vi "Laser Power Control.vi"(7 "Calling VI Ref":refnum<vi>) -> ()   [LabVIEW 2020]
uses:
  Laser Power Control Type Defs/Laser Power Ctrl Main Control.ctl
  Laser Power Control Type Defs/Laser Power Ctrl Setup.ctl
  Hardware Configuration/Hardware Configuration Controls/Device Type.ctl
  <vilib>/Utility/miscctls.llb/LVPointTypeDef.ctl
  Laser Power Control Type Defs/Laser Power Ctrl Settings.ctl
  Hardware Configuration/Hardware Configuration Controls/Device Function.ctl
  Laser Power Control Type Defs/Laser Power Ctrl Notifier Type.ctl
  Laser Power Control Type Defs/Laser Power Ctrl Actions.ctl
  Laser Power Control Type Defs/Laser Power Ctrl Base Type.ctl
  Laser Power Control Type Defs/Laser Power Ctrl Type.ctl
  Device Library/Lasers/Laser Controls/Laser Actions.ctl
  Device Library/AOTFs/AOTF Controls/AOTF Actions.ctl
  Device Library/Lasers/External Power Control/External Power Control Type Defs/External Power Actions.ctl
  Device Manager/Common Device Queue/Common Device Controls/Common Device Actions.ctl
  <vilib>/regexp/Match Regular Expression.xnode
panel:
  in  "Manual Laser Ctrl.":bool
  out "Tab Control":enum32{"Power Adjust", "Setup"}(tab)
  in  "Power Ctrl 04":T1={"Wavelength (nm)"=0, "Active"=TRUE, "Power"=0.0, "Power Slider"=0, "Ctrl Status"=""} {"Power Slider" scale=0.0..100.0}
  in  "Power Ctrl 03":T1={"Wavelength (nm)"=0, "Active"=TRUE, "Power"=0.0, "Power Slider"=0, "Ctrl Status"=""} {"Power Slider" scale=0.0..100.0}
  in  "Power Ctrl 02":T1={"Wavelength (nm)"=0, "Active"=TRUE, "Power"=0.0, "Power Slider"=0, "Ctrl Status"=""} {"Power Slider" scale=0.0..100.0}
  in  "Power Ctrl 01":T1={"Wavelength (nm)"=0, "Active"=TRUE, "Power"=0.0, "Power Slider"=0, "Ctrl Status"=""} {"Power Slider" scale=0.0..100.0}
  in  "Power Ctrl 00":T1={"Wavelength (nm)"=0, "Active"=TRUE, "Power"=0.0, "Power Slider"=0, "Ctrl Status"=""} {"Power Slider" scale=0.0..100.0}
  in  "Power Setup 04":T2 {"Power Control Mode" items=["Direct", "AOTF", "External Ctrl", "Ext + AOTF"]}
  in  "Power Setup 03":T2 {"Power Control Mode" items=["Direct", "AOTF", "External Ctrl", "Ext + AOTF"]}
  in  "Power Setup 02":T2 {"Power Control Mode" items=["Direct", "AOTF", "External Ctrl", "Ext + AOTF"]}
  in  "Power Setup 01":T2 {"Power Control Mode" items=["Direct", "AOTF", "External Ctrl", "Ext + AOTF"]}
  in  "Power Setup 00":T2 {"Power Control Mode" items=["Direct", "AOTF", "External Ctrl", "Ext + AOTF"]}
  in  "Power Ctrl Setup":bool=TRUE
  in  "Quit":bool
  # "Ctrl Status:"
  # "Ctrl Status:"
  # "Ctrl Status:"
  # "Ctrl Status:"
  # "Ctrl Status:"
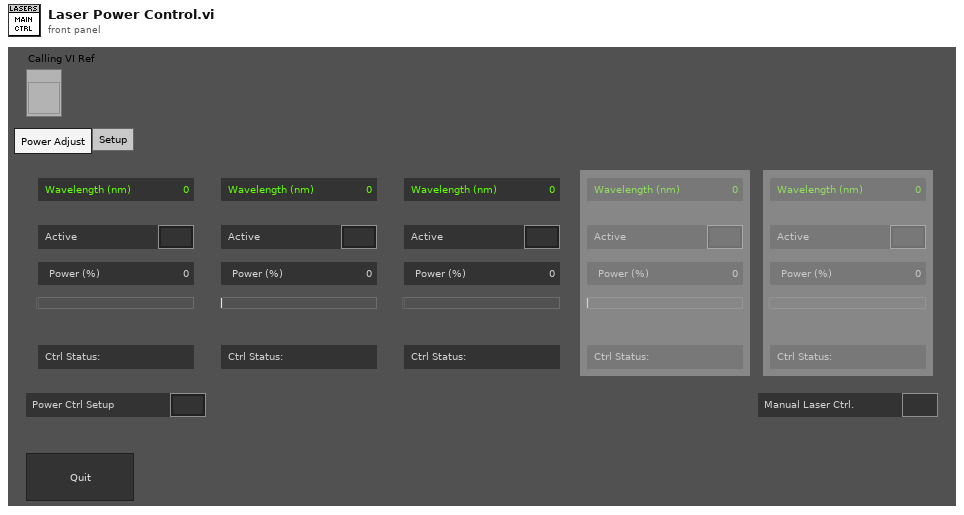
[diagram p1: front panel]
types:
  T1 = typedef "Laser Power Ctrl Main Control.ctl" = cluster{"Wavelength (nm)":u16, "Active":bool, "Power":dbl, "Power Slider":u8, "Ctrl Status":string}
  T2 = typedef "Laser Power Ctrl Setup.ctl" = cluster{"Wavelength (nm)":u16, "Power Control Mode":u16, "Ext Settings":bool, "Ext. Ctrl":string, "Pop Out":bool}
  T3 = typedef "Device Function.ctl" = enum16{"Primary", "Secondary", "Overview", "Wide Field Drift Correction", "642 nm Excitation", "560 nm Excitation", "940 nm Excitation", "546 nm Excitation", "488 nm Excitation", "405 nm Excitation", "Objective Drift Correction", "4Pi Objective Lock", "Objective XY", "Objective Z", "Sample XY", "Sample Coarse Z", "Sample Z", "4Pi Lower", "4Pi Upper", "Mojo", "Adj Cavity", "Line Scanning", "Alert"}
  T4 = typedef "Device Type.ctl" = enum16{"AOTF", "Camera", "Deformable Mirror", "Laser", "Microscope Base", "Shutter", "Stage", "Waveform", "FPGA", "Email", "Filter Wheel", "Spinning Disk"}
  T5 = typedef "Laser Power Ctrl Settings.ctl" = cluster{"Wavelength":u16, "Ctrl Mode":u16, "Ext Ctrl Path":string, "Settings":string[]}
  T6 = enum16{"Always On", "Always Off", "Off While Running"}
  T7 = typedef "LVPointTypeDef.ctl" = cluster{"Horizontal":i16, "Vertical":i16}
  T8 = typedef "LVRectTypeDef.ctl" = cluster{"Left":i16, "Top":i16, "Right":i16, "Bottom":i16}
  T9 = typedef "LVBoundsTypeDef.ctl" = cluster{"Width":u32, "Height":u32}
  T10 = typedef "Laser Power Ctrl Base Type.ctl" = cluster{"Active":bool, "Power":dbl, "Ctrl Mode":u16}
  T11 = typedef "Laser Power Ctrl Actions.ctl" = enum16{"Exit Loop", "Active", "Power Adj", "All Active On", "All Active Off", "Quit"}
  T12 = typedef "Laser Power Ctrl Notifier Type.ctl" = cluster{"Actions":T11, "Wavelength":u16, "Wavelengths":u16[], "Power Ctrl":T10[]}
  T13 = typedef "Laser Actions.ctl" = enum16{"Error Check", "Set On/Off", "Set Power", "Set Parameter", "Get Power", "Get Status", "Get Parameter", "Quit"}
  T14 = typedef "AOTF Actions.ctl" = enum16{"Error Check", "Blank", "Line On/Off", "Set Power", "Status", "Quit"}
  T15 = typedef "External Power Actions.ctl" = enum16{"Line On/Off", "Set Power", "Set Ctrl Parameters", "Quit"}
  T16 = enum8{"Enabled", "Disabled", "Disabled and Grayed Out"}
  T17 = typedef "Laser Power Ctrl Type.ctl" = enum16{"Direct", "AOTF", "Ext Control"}
  T18 = typedef "Common Device Actions.ctl" = enum16{"Specific Action", "Open Front Panel", "Close Front Panel", "Quit", "Quit All"}
  T19 = cluster{"Wavelength (nm)":bool, "Active":bool, "Power":bool, "Power Slider":bool, "Ctrl Status":bool}
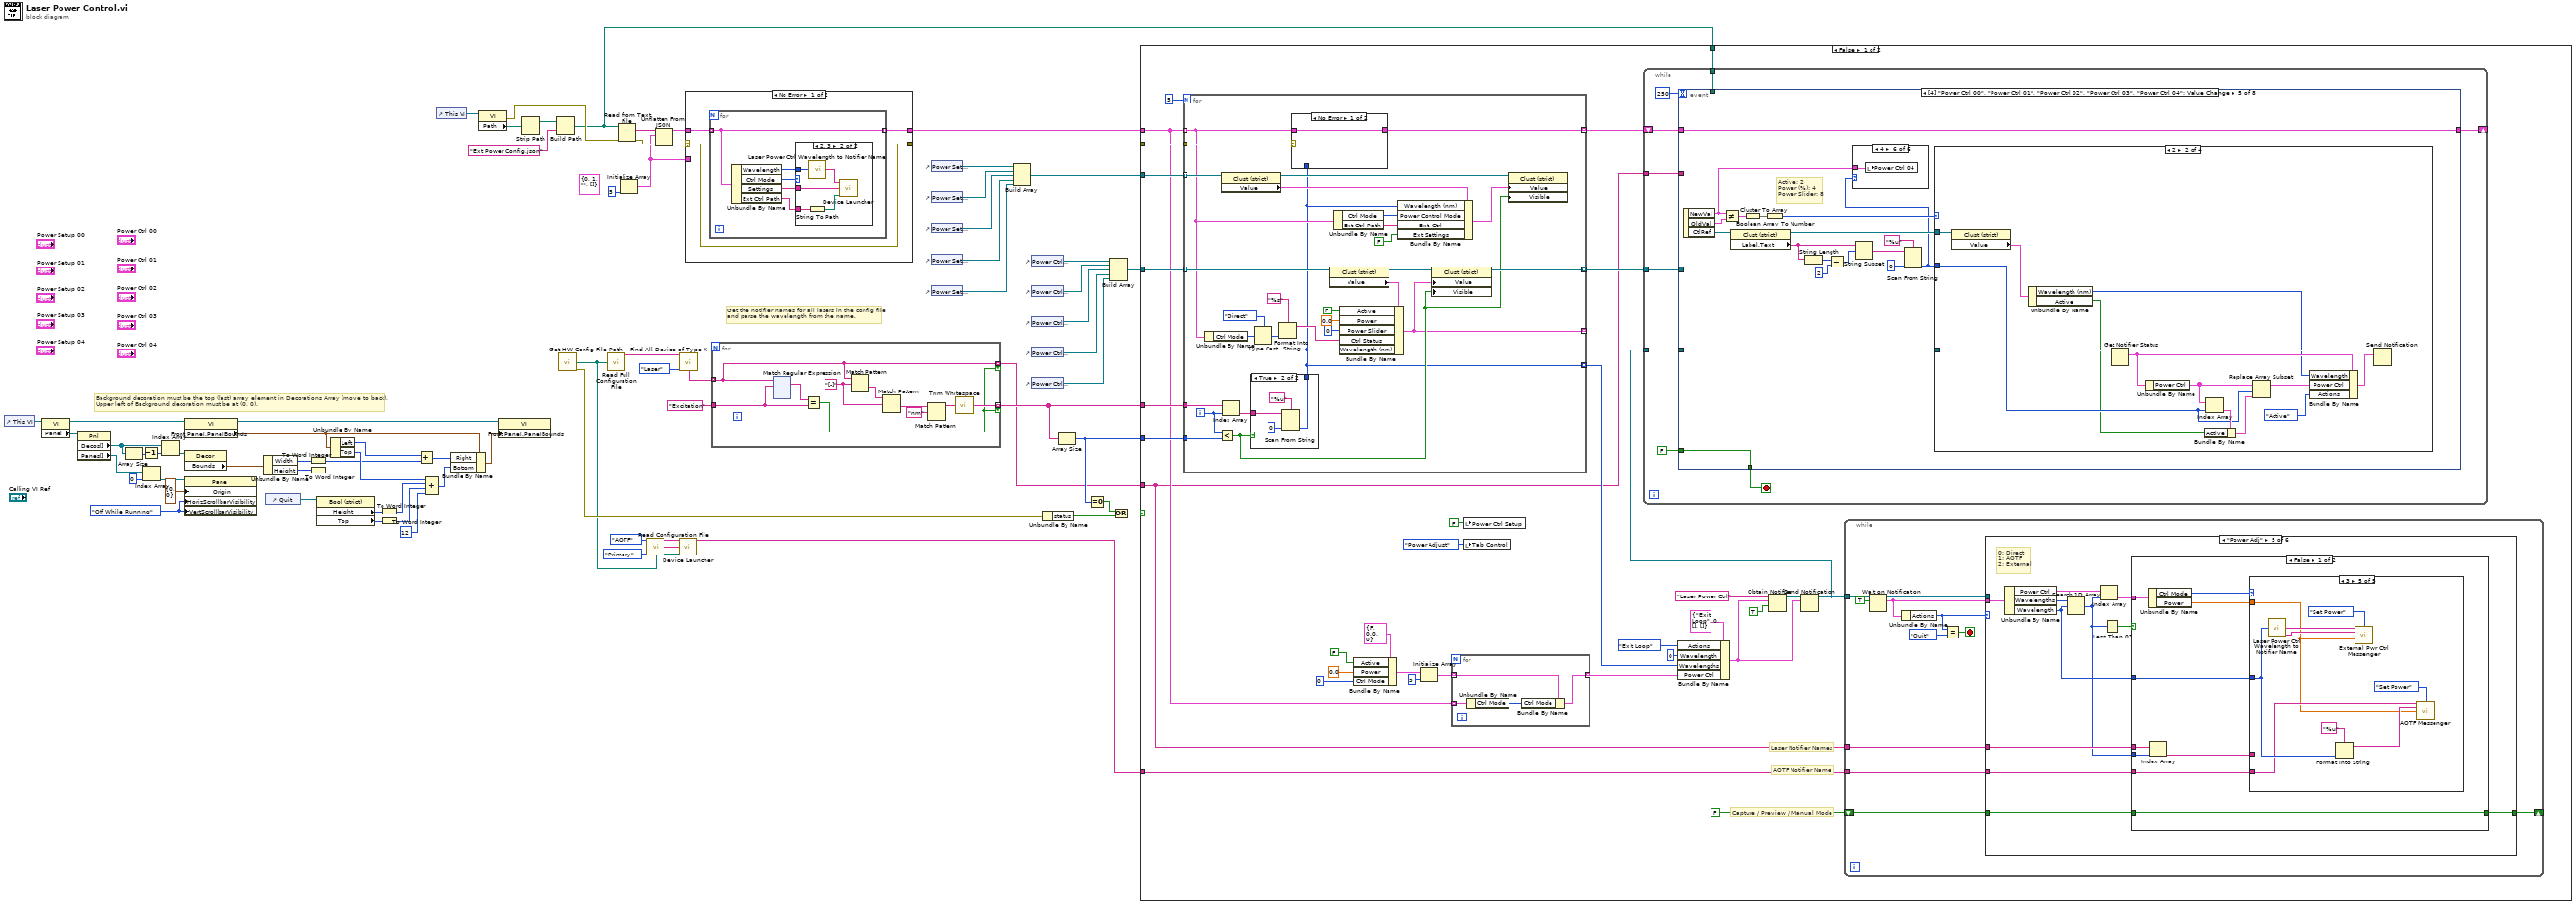
[diagram p0: block diagram]
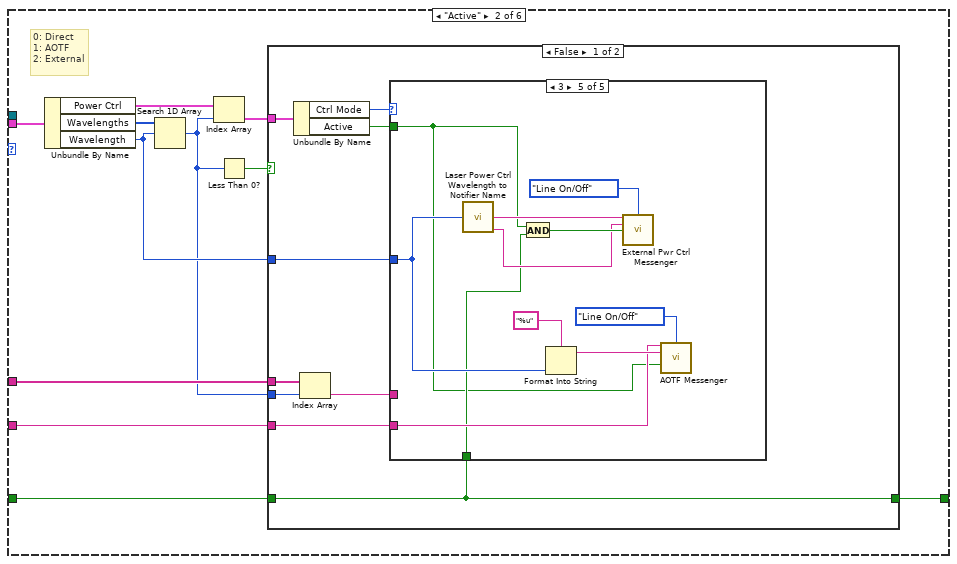
[diagram p5: hidden frame]
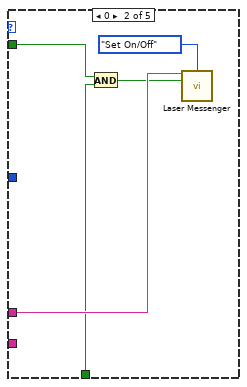
[diagram p7: hidden frame]
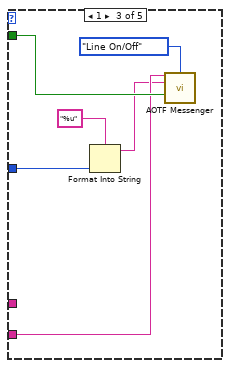
[diagram p8: hidden frame]
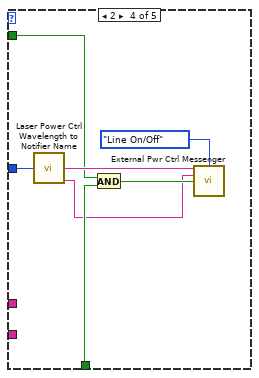
[diagram p9: hidden frame]
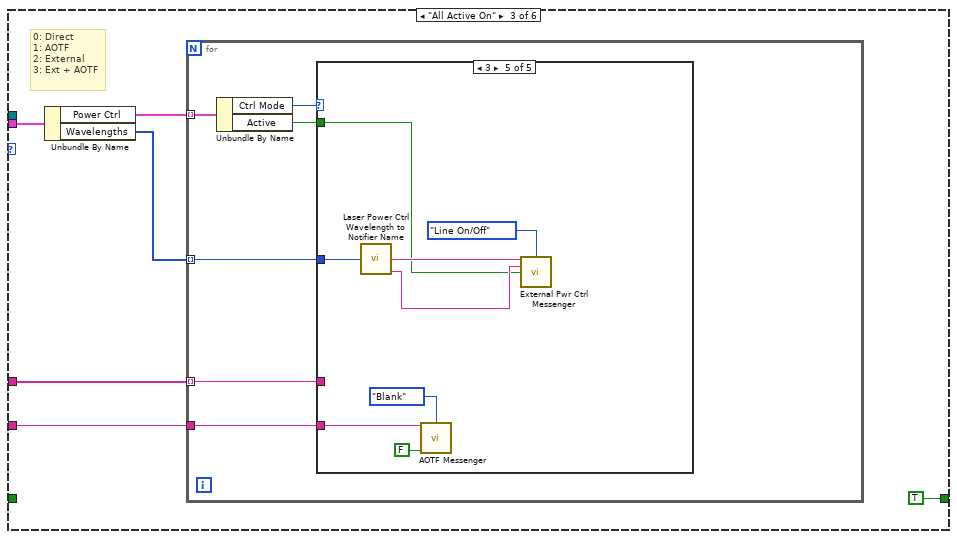
[diagram p11: hidden frame]
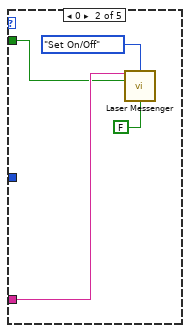
[diagram p13: hidden frame]
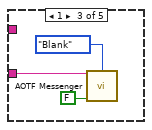
[diagram p14: hidden frame]
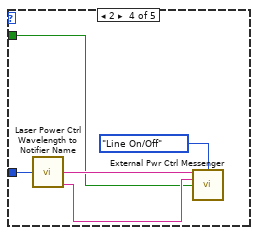
[diagram p15: hidden frame]
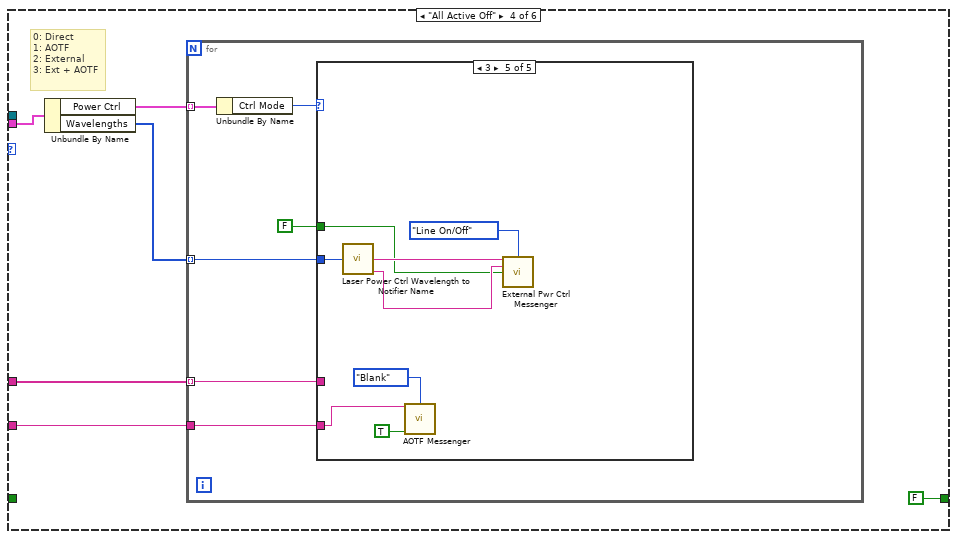
[diagram p16: hidden frame]
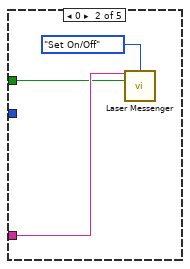
[diagram p18: hidden frame]
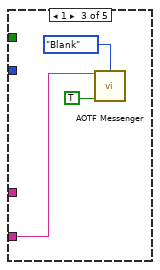
[diagram p19: hidden frame]
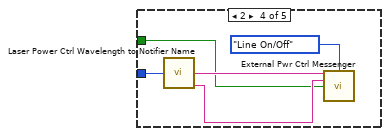
[diagram p20: hidden frame]
diagram:
  w55 = T6."Off While Running" ("Vertical Scrollbar Visibility")
  # "Get the notifier names for all lasers in the config file\nand parse the wavelength from the name."
  # "Background decoration must be the top (last) array element in Decorations Array (move to back).\nUpper left of Background decoration must be at (0, 0)."
  n1 = control-ref of="This VI"() -> (w47:refnum<vi>)
  n2 = property class="VI"(reference=w47) -> (reference out=w56:refnum<vi>, "Panel"=w48:refnum<vi>)  [unwired: 1 in, 1 out]
  n3 = property class="Pnl"(reference=w48) -> ("Decos[]"=w46:refnum<vi>[], "Panes[]"=w52:refnum<vi>[])  [unwired: 1 in, 2 out]
  n4 = Array Size(array=w46) -> (size(s)=w44:i32)
  n5 = Decrement(x=w44) -> (x-1=w45:i32)
  n6 = Index Array(array=w52, index=0) -> (element=w51:refnum<vi>)
  n7 = Index Array(array=w46, index=w45) -> (element=w54:refnum<vi>)
  n8 = property class="VI"(reference=w56) -> (reference out=w58:refnum<vi>, "Front Panel.PanelBounds"=w59:T8)  [unwired: 1 in, 1 out]
  n9 = property class="Decor"(reference=w54) -> ("Bounds"=w57:T9)  [unwired: 1 in, 2 out]
  n10 = property class="Pane"(reference=w51, "Origin"=T7 {"Horizontal"=0, "Vertical"=0}, "HorizScrollbarVisibility"=w55, "VertScrollbarVisibility"=w55) -> ()  [unwired: 1 in, 2 out]
  n11 = Unbundle By Name(w57) -> ("Width"=w62:u32, "Height"=w65:u32)
  n12 = control-ref of="Quit"() -> (w49:refnum<vi>)
  n13 = To Word Integer(number=w62) -> (16bit integer=w64:i16)
  n14 = To Word Integer(number=w65) -> ()  [unwired: 1 out]
  n15 = property class="Bool (strict)"(reference=w49) -> ("Height"=w67:u32, "Top"=w68:i32)  [unwired: 1 in, 2 out]
  n16 = Unbundle By Name(w59) -> ("Left"=w61:i16, "Top"=w72:i16)
  n17 = To Word Integer(number=w67) -> (16bit integer=w70:i16)
  n18 = To Word Integer(number=w68) -> (16bit integer=w71:i16)
  n19 = Add(x=w61, y=w64) -> (x+y=w63:i16)
  n20 = Compound Arithmetic op=ADD(w72, w70, w71, i16 12 ("y")) -> (w66:i16)
  n21 = control-ref of="This VI"() -> (w23:refnum<vi>)
  n22 = Bundle By Name(cluster=w59, "Right"=w63, "Bottom"=w66) -> (w60:T8)
  n23 = property class="VI"(reference=w23) -> (error out=w16:errorcluster, "Path"=w22:path)  [unwired: 1 in, 1 out]
  n24 = property class="VI"(reference=w58, "Front Panel.PanelBounds"=w60) -> ()  [unwired: 1 in, 2 out]
  n25 = Strip Path(path=w22) -> (stripped path=w21:path)  [unwired: 1 out]
  n26 = Build Path(base path=w21, name or relative path="Ext Power Config.json") -> (appended path=w1:path)
  n27 = call "Get HW Config File Path.vi"() -> ("File Path"=w6:path, "Error"=w39:errorcluster)  [unwired: 14 in]
  n28 = call "Read Full Configuration File.vi"("Config File Path"=w6) -> ("Unique Notifier Names"=w74:string[])  [unwired: 11 in, 3 out]
  n29 = Read from Text File(file (use dialog)=w1, error in=w16) -> (text=w19:string, error out=w18:errorcluster)  [unwired: 2 in, 2 out]
  n30 = Initialize Array(T5 {"Wavelength"=0, "Ctrl Mode"=1, "Ext Ctrl Path"="", "Settings"=[]} ("Power Ctrl Settings"), 5 ("dimension size")) -> (w12:T5[])
  n31 = call "Read Configuration File.vi"("Device Type"=Device_Type."AOTF", "Device Function"=Device_Function."Primary", "Config File Path"=w6) -> ("Unique Notifier Name"=w5:string, "Device Ports/IDs/Channels"=w4:string[], "Device Engine Path"=w3:path)  [unwired: 9 in, 1 out]
  n32 = Unflatten From JSON(JSON string=w19, type and defaults=w12, error in (no error)=w18) -> (value=w15:T5[], error out=w17:errorcluster)  [unwired: 4 in]
  n33 = call "Device Launcher.vi"("Notifier Name"=w5, "Device Ports/IDs/Channels"=w4, "Device Engine Path"=w3) -> ("Notifier Name"=w2:string)  [unwired: 11 in, 1 out]
  n34 = call "Find All Device of Type X.vi"("Unique Notifier Names"=w74, "Device Type"=Device_Type."Laser") -> ("All Devices"=w43:string[])  [unwired: 12 in, 1 out]
  n35 = case shown="No Error" w17 {
    selector: w17 -> [w75 w88]
    tunnel: w15 -> [w77 _]
    tunnel: [w76 w89] -> w11
    tunnel: w12 -> [_ w89]
    tunnel: [w75 w88] -> w10
    frame No Error {
      n36 = for {
        tunnel: w77 -> [w82] mode=indexing
        tunnel: [w82] -> w76 mode=indexing
        n37 = Unbundle By Name(w82) -> ("Wavelength"=w80:u16, "Ctrl Mode"=w81:u16, "Settings"=w79:string[], "Ext Ctrl Path"=w78:string)
        n38 = case shown="2, 3" w81 {
          tunnel: w80 -> [_ w84]
          tunnel: w79 -> [_ w87]
          tunnel: w78 -> [_ w86]
          frame Default {
          }
          frame 2, 3 {
            n39 = String To Path(string=w86) -> (path=w85:path)
            n40 = call "Laser Power Ctrl Wavelength to Notifier Name.vi"("Wavelength"=w84) -> ("Notifier Name"=w83:string)  [unwired: 13 in, 1 out]
            n41 = call "Device Launcher.vi"("Notifier Name"=w83, "Device Ports/IDs/Channels"=w87, "Device Engine Path"=w85) -> ()  [unwired: 11 in, 2 out]
          }
        }
      }
    }
    frame Error {
    }
  }
  n42 = for {
    tunnel: w43 -> [w97] mode=indexing
    tunnel: [w97] -> w35 mode=indexing if=w90
    tunnel: "Excitation" -> [w98]
    tunnel: [w91] -> w37 mode=indexing if=w90
    w95 = "[-]" ("regular expression")
    n43 = xnode "Match Regular Expression"("input string"=w97, "regular expression"=w98) -> ("whole match"=w99:string)  [unwired: 4 in, 4 out]
    n44 = Equal?(x=w99, y=w98) -> (x = y?=w90:bool)
    n45 = Match Pattern(string=w97, regular expression=w95) -> (after substring=w96:string)  [unwired: 1 in, 3 out]
    n46 = Match Pattern(string=w96, regular expression=w95) -> (after substring=w94:string)  [unwired: 1 in, 3 out]
    n47 = Match Pattern(string=w94, regular expression="nm") -> (before substring=w92:string)  [unwired: 1 in, 3 out]
    n48 = call <vilib>:"Trim Whitespace.vi"("string"=w92) -> ("trimmed string"=w91:string)  [unwired: 1 in]
  }
  n49 = control-ref of="Power Setup 00"() -> (w28:refnum<vi>)
  n50 = control-ref of="Power Setup 01"() -> (w24:refnum<vi>)
  n51 = control-ref of="Power Setup 02"() -> (w25:refnum<vi>)
  n52 = control-ref of="Power Setup 03"() -> (w26:refnum<vi>)
  n53 = control-ref of="Power Setup 04"() -> (w27:refnum<vi>)
  n54 = Build Array(w28, w24, w25, w26, w27) -> (w9:refnum<vi>[])
  n55 = control-ref of="Power Ctrl 00"() -> (w30:refnum<vi>)
  n56 = control-ref of="Power Ctrl 01"() -> (w31:refnum<vi>)
  n57 = control-ref of="Power Ctrl 02"() -> (w32:refnum<vi>)
  n58 = control-ref of="Power Ctrl 03"() -> (w33:refnum<vi>)
  n59 = control-ref of="Power Ctrl 04"() -> (w34:refnum<vi>)
  n60 = Unbundle By Name(w39) -> ("status"=w38:bool)
  n61 = Array Size(array=w37) -> (size(s)=w41:i32)
  n62 = Equal To 0?(x=w41) -> (x = 0?=w40:bool)
  n63 = Build Array(w30, w31, w32, w33, w34) -> (w29:refnum<vi>[])
  n64 = Or(x=w40, y=w38) -> (x .or. y?=w36:bool)
  n65 = case shown="False" w36 {
    tunnel: w41 -> [w245 _]
    tunnel: w37 -> [w244 _]
    tunnel: w35 -> [w218 _]
    tunnel: w29 -> [w242 _]
    tunnel: w9 -> [w241 _]
    tunnel: w11 -> [w225 _]
    tunnel: w10 -> [w240 _]
    tunnel: w2 -> [w219 _]
    tunnel: w1 -> [w214 _]
    frame False {
      # "AOTF Notifier Name"
      # "Laser Notifier Names"
      # "Capture / Preview / Manual Mode"
      n66 = for {
        N: 5 -> [_]
        tunnel: w244 -> [w825]
        tunnel: [w826] -> w243 mode=indexing
        tunnel: w245 -> [w823]
        tunnel: w242 -> [w821] mode=indexing
        tunnel: w241 -> [w815] mode=indexing
        tunnel: w225 -> [w805] mode=indexing
        tunnel: w240 -> [w806]
        tunnel: [w810] -> w221 mode=indexing
        tunnel: [w799] -> _ mode=indexing
        tunnel: [w798] -> w226 mode=indexing
        i -> [w824]
        n67 = Unbundle By Name(w805) -> ("Ctrl Mode"=w800:u16)
        n68 = Less?(x=w824, y=w823) -> (x < y?=w811:bool)
        n69 = property class="Clust (strict)"(reference=w815) -> (reference out=w813:refnum<vi>, "Value"=w814:T2)  [unwired: 1 in, 1 out]
        n70 = Index Array(array=w825, index=w824) -> (element=w822:string)
        n71 = case shown="True" w811 {
          tunnel: [u16 0 ("default value 1") w833] -> w798
          tunnel: w822 -> [_ w832]
          frame False {
          }
          frame True {
            n72 = Scan From String(format string="%u", input string=w832, default 1=u16 0 ("default value 1")) -> (output 1=w833:u16)  [unwired: 2 in, 3 out]
          }
        }
        n73 = Type Cast(type=Laser_Power_Ctrl_Type."Direct" ("Control Mode"), x=w800) -> (*(type *) &x=w802:T17)
        n74 = Format Into String(format string="%s", w802) -> (resulting string=w804:string)  [unwired: 2 in, 1 out]
        n75 = case shown="No Error" w806 {
          tunnel: w805 -> [w827 w830]
          tunnel: w798 -> [_ w829]
          tunnel: [w827 w828] -> w810
          frame No Error {
          }
          frame Error {
            n76 = Bundle By Name(cluster=w830, "Wavelength"=w829) -> (w828:T5)
          }
        }
        n77 = property class="Clust (strict)"(reference=w821) -> (reference out=w820:refnum<vi>, "Value"=w819:T1)  [unwired: 1 in, 1 out]
        n78 = Unbundle By Name(w805) -> ("Ctrl Mode"=w809:u16, "Ext Ctrl Path"=w808:string)
        n79 = Bundle By Name(cluster=w819, "Active"=FALSE, "Power"=0.0 ("Power (%)"), "Power Slider"=u8 0, "Ctrl Status"=w804, "Wavelength (nm)"=w798) -> (w799:T1)
        n80 = Bundle By Name(cluster=w814, "Wavelength (nm)"=w798, "Power Control Mode"=w809, "Ext. Ctrl"=w808, "Ext Settings"=FALSE) -> (w812:T2)
        n81 = property class="Clust (strict)"(reference=w820, "Value"=w799, "Visible"=w811) -> (reference out=w826:refnum<vi>)  [unwired: 1 in, 1 out]
        n82 = property class="Clust (strict)"(reference=w813, "Value"=w812, "Visible"=w811) -> ()  [unwired: 1 in, 2 out]
      }
      n83 = Bundle By Name(cluster=T10 {"Active"=FALSE, "Power"=0.0, "Ctrl Mode"=0} ("Power Ctrl"), "Active"=FALSE, "Power"=0.0, "Ctrl Mode"=u16 0) -> (w229:T10)
      n84 = Initialize Array(w229, 5 ("dimension size")) -> (w224:T10[])
      n85 = for {
        tunnel: w225 -> [w249] mode=indexing
        tunnel: w224 -> [w248] mode=indexing
        tunnel: [w246] -> w223 mode=indexing
        n86 = Unbundle By Name(w249) -> ("Ctrl Mode"=w247:u16)
        n87 = Bundle By Name(cluster=w248, "Ctrl Mode"=w247) -> (w246:T10)
      }
      n88 = local write "Power Ctrl Setup"(FALSE ("Power Ctrl Setup")) -> ()
      n89 = local write "Tab Control"(enum32{"Power Adjust", "Setup"}."Power Adjust" ("Tab Control")) -> ()
      n90 = Bundle By Name(cluster=T12 {"Actions"=enum."Exit Loop", "Wavelength"=0, "Wavelengths"=[], "Power Ctrl"=[]} ("Laser Power Ctrl Note Type"), "Actions"=Laser_Power_Ctrl_Actions."Exit Loop", "Wavelength"=u16 0 ("Index"), "Wavelengths"=w226, "Power Ctrl"=w223) -> (w233:T12)
      n91 = Obtain Notifier(name (unnamed)="Laser Power Ctrl", notification data type=w233, create if not found? (T)=TRUE) -> (notifier out=w239:refnum<notifier>)  [unwired: 1 in, 2 out]
      n92 = Send Notification(notification=w233, notifier=w239) -> (notifier out=w232:refnum<notifier>)  [unwired: 1 in, 1 out]
      n93 = while {
        tunnel: w243 -> [w428]
        tunnel: w232 -> [w425]
        shift-right: [w423] -> _
        shift-left: w221 -> [w424]
        tunnel: w218 -> [w422]
        tunnel: w214 -> [w421]
        stop <- w427 stop-if-true
        n94 = event shown="[4] \"Power Ctrl 00\", \"Power Ctrl 01\", \"Power Ctrl 02\", \"Power Ctrl 03\", \"Power Ctrl 04\": Value Change" {
          selector: _ -> [_ _ _ _ _ _ _ _]
          dyn-events: _ -> [_ _ _ _ _ _ _ _]
          timeout: 250 -> [_ _ _ _ _ _ _ _]
          tunnel: w428 -> [w434 w465 _ _ _ _ _ _]
          tunnel: [w436 w490 w646 w682 w700 w763 w769 w786] -> w427
          tunnel: FALSE -> [w436 w490 w646 w682 w700 w763 w769 _]
          tunnel: w425 -> [w433 w457 _ _ w685 w760 _ w785]
          tunnel: w424 -> [w435 w477 w643 w680 w691 w762 w764 w771]
          tunnel: [w435 w474 w639 w680 w691 w762 w764 w771] -> w423
          tunnel: w422 -> [w430 w456 _ _ _ _ _ _]
          tunnel: w421 -> [_ _ _ _ _ _ _ w770]
          event Timeout {
            # "Monitor power for case with direct control (from laser) and for % ctrl (in case outside apps change the power)"
            n95 = event-data() -> ()  [unwired: 1 in, 1 out]
            n96 = Get Notifier Status(notifier=w433) -> (current notification=w432:T12)  [unwired: 1 in, 4 out]
            n97 = Unbundle By Name(w432) -> ("Power Ctrl"=w431:T10[])
            n98 = for {
              tunnel: w434 -> [w451] mode=indexing
              tunnel: w431 -> [w449] mode=indexing
              tunnel: w430 -> [w442] mode=indexing
              n99 = Unbundle By Name(w449) -> ("Active"=w448:bool, "Power"=w444:dbl, "Ctrl Mode"=w446:u16)
              n100 = property class="Clust (strict)"(reference=w451) -> (reference out=w441:refnum<vi>, "Value"=w450:T1)  [unwired: 1 in, 1 out]
              n101 = case shown="1, 2, Default" w446 {
                tunnel: [0.0 w453] -> w445
                tunnel: w444 -> [_ w453]
                frame 0 {
                }
                frame 1, 2, Default {
                }
              }
              n102 = call "Device Manager Check if Running.vi"("Notifier Name"=w442) -> ("Running?"=w440:bool)  [unwired: 14 in]
              n103 = To Unsigned Byte Integer(number=w445) -> (unsigned 8bit integer=w447:u8)
              n104 = Select(t=T16."Enabled" ("Disabled"), s=w440, f=T16."Disabled and Grayed Out" ("Disabled")) -> (s? t:f=w437:T16)
              n105 = Bundle By Name(cluster=w450, "Active"=w448, "Power"=w445, "Power Slider"=w447) -> (w443:T1)
              n106 = property class="Clust (strict)"(reference=w441, "DisabledEnum"=w437, "Value"=w443) -> ()  [unwired: 1 in, 2 out]
            }
          }
          event Value Change {
            w473 = refnum<vi> refnum  # Generic
            w489 = refnum<vi> refnum  # Generic
            # "This got messy..."
            # "0: Direct\n1: AOTF\n2: External\n3: Ext + AOTF"
            n107 = event-data() -> ("CtlRef"=w478:refnum<vi>, "NewVal"=w480:u16)  [unwired: 1 in]
            n108 = To More Generic Class(target class=w489, reference=w478) -> (generic class reference=w488:refnum<vi>)
            n109 = call "Laser Power Ctrl Index from Name.vi"("Generic Class Ref"=w488) -> ("Index from Name"=w454:i32)  [unwired: 14 in]
            n110 = Index Array(array=w465, index=w454) -> (element=w455:refnum<vi>)
            n111 = Get Notifier Status(notifier=w457) -> (notifier out=w487:refnum<notifier>, current notification=w484:T12)  [unwired: 1 in, 3 out]
            n112 = Index Array(array=w477, index=w454) -> (element=w476:T5)
            n113 = Unbundle By Name(w484) -> ("Power Ctrl"=w482:T10[])
            n114 = case shown="3" w480 {
              selector: w480 -> [w513 w520 _ _]
              tunnel: w478 -> [w510 w523 w529 w575]
              tunnel: w476 -> [w517 w518 w531 w577]
              tunnel: [w516 w524 w530 w576] -> w475
              tunnel: [w510 w523 w529 w575] -> w471
              tunnel: [FALSE FALSE w528 w574] -> w472
              tunnel: [path "" path "" w527 w573] -> w469
              tunnel: [w513 w520 w526 w572] -> w463
              tunnel: ["Power (mW)" "Power (%)" w525 w571] -> w459
              tunnel: w456 -> [w502 _ _ _]
              tunnel: w455 -> [w500 _ _ _]
              tunnel: w454 -> [w496 _ _ _]
              frame 0, Default {
                w494 = refnum<vi> refnum  # Boolean
                (unwired) refnum<vi> refnum  # Cluster
                w499 = refnum<vi> refnum  # Cluster
                # "Not sure why, but this wont set the value..."
                n115 = Index Array(array=w502, index=w496) -> (element=w501:string)
                n116 = property class="Ring (strict)"(reference=w510) -> ("Owner"=w511:refnum<vi>)  [unwired: 1 in, 2 out]
                n117 = property class="Clust (strict)"(reference=w500) -> ("Controls[]"=w497:refnum<vi>[])  [unwired: 1 in, 2 out]
                n118 = To More Specific Class(target class=w499, reference=w511) -> (specific class reference=w509:refnum<vi>)  [unwired: 1 in, 1 out]
                n119 = property class="Clust"(reference=w509) -> ("Controls[]"=w508:refnum<vi>[])  [unwired: 1 in, 2 out]
                n120 = call "Laser Messenger.vi"("Notifier Name"=w501, "Action"=Laser_Actions."Get Status") -> ("Light Emission?"=w491:bool)  [unwired: 8 in, 5 out]
                n121 = To Variant(anything=w491) -> (Variant=w492:variant)
                n122 = Index Array(array=w508, index=4) -> (element=w506:refnum<vi>)
                n123 = To Variant(anything=TRUE) -> (Variant=w505:variant)
                n124 = property class="Ctl"(reference=w506, "Value"=w505) -> ()  [unwired: 1 in, 2 out]
                n125 = Index Array(array=w497, index=1) -> (element=w495:refnum<vi>)
                n126 = To More Specific Class(target class=w494, reference=w495) -> (specific class reference=w493:refnum<vi>)  [unwired: 1 in, 1 out]
                n127 = property class="Bool"(reference=w493, "Value"=w492) -> ()  [unwired: 1 in, 2 out]
                n128 = Bundle By Name(cluster=w517, "Ctrl Mode"=w513) -> (w516:T5)
              }
              frame 1 {
                # "AOTF"
                n129 = Bundle By Name(cluster=w518, "Ctrl Mode"=w520) -> (w524:T5)
              }
              frame 2 {
                n130 = Unbundle By Name(w531) -> ("Wavelength"=w534:u16, "Ext Ctrl Path"=w541:string, "Settings"=w539:string[])
                n131 = call "Laser Power Ctrl Wavelength to Notifier Name.vi"("Wavelength"=w534) -> ("Notifier Name"=w533:string)  [unwired: 13 in, 1 out]
                n132 = call "Device Manager Check if Running.vi"("Notifier Name"=w533) -> ("Running?"=w543:bool)  [unwired: 14 in]
                n133 = case shown="True" w543 {
                  tunnel: w534 -> [w564 w570]
                  tunnel: [w564 w570] -> w542
                  tunnel: w541 -> [w563 w569]
                  tunnel: [w563 w569] -> w540
                  tunnel: w539 -> [w562 w568]
                  tunnel: [w562 w568] -> w538
                  tunnel: w533 -> [w561 w566]
                  tunnel: [w561 w565] -> w536
                  frame False {
                  }
                  frame True {
                    n134 = call "Common Device Queue Messenger.vi"("Common Action"=Common_Device_Actions."Quit" ("Common Actions"), "Notifier Name"=w566) -> ("Notifier Name"=w565:string)  [unwired: 13 in]
                  }
                }
                n135 = String To Path(string=w540) -> (path=w544:path)
                n136 = call "Laser Power Ctrl Ext Setup.vi"("Wavelength"=w542, "Previous Path"=w544, "Settings"=w538) -> ("Settings Out"=w532:string[], "Ext Ctrl Path"=w537:path, "Canceled?"=w535:bool)  [unwired: 10 in]
                n137 = case shown="False" w535 {
                  tunnel: w537 -> [w547 _]
                  tunnel: w532 -> [w550 _]
                  tunnel: w536 -> [w554 _]
                  tunnel: w529 -> [_ w560]
                  tunnel: [TRUE FALSE] -> w528
                  tunnel: w531 -> [w549 w558]
                  tunnel: [w548 w558] -> w530
                  tunnel: [w547 path ""] -> w527
                  tunnel: [u16 2 ("Ctrl Mode") w556] -> w526
                  tunnel: ["Power (%)" "Power (%)"] -> w525
                  frame False {
                    n138 = Path To String(path=w547) -> (string=w551:string)
                    n139 = call "Device Launcher.vi"("Notifier Name"=w554, "Device Ports/IDs/Channels"=w550, "Device Engine Path"=w547) -> ()  [unwired: 11 in, 2 out]
                    n140 = Bundle By Name(cluster=w549, "Ctrl Mode"=u16 2, "Settings"=w550, "Ext Ctrl Path"=w551) -> (w548:T5)
                  }
                  frame True {
                    w556 = u16 1 ("Value")
                    n141 = property class="Ring (strict)"(reference=w560, "Value"=w556) -> ()  [unwired: 1 in, 2 out]
                  }
                }
              }
              frame 3 {
                n142 = Unbundle By Name(w577) -> ("Wavelength"=w580:u16, "Ext Ctrl Path"=w587:string, "Settings"=w585:string[])
                n143 = call "Laser Power Ctrl Wavelength to Notifier Name.vi"("Wavelength"=w580) -> ("Notifier Name"=w579:string)  [unwired: 13 in, 1 out]
                n144 = call "Device Manager Check if Running.vi"("Notifier Name"=w579) -> ("Running?"=w589:bool)  [unwired: 14 in]
                n145 = case shown="True" w589 {
                  tunnel: w580 -> [w610 w616]
                  tunnel: [w610 w616] -> w588
                  tunnel: w587 -> [w609 w615]
                  tunnel: [w609 w615] -> w586
                  tunnel: w585 -> [w608 w614]
                  tunnel: [w608 w614] -> w584
                  tunnel: w579 -> [w607 w612]
                  tunnel: [w607 w611] -> w582
                  frame False {
                  }
                  frame True {
                    n146 = call "Common Device Queue Messenger.vi"("Common Action"=Common_Device_Actions."Quit" ("Common Actions"), "Notifier Name"=w612) -> ("Notifier Name"=w611:string)  [unwired: 13 in]
                  }
                }
                n147 = String To Path(string=w586) -> (path=w590:path)
                n148 = call "Laser Power Ctrl Ext Setup.vi"("Wavelength"=w588, "Previous Path"=w590, "Settings"=w584) -> ("Settings Out"=w578:string[], "Ext Ctrl Path"=w583:path, "Canceled?"=w581:bool)  [unwired: 10 in]
                n149 = case shown="False" w581 {
                  tunnel: w583 -> [w593 _]
                  tunnel: w578 -> [w596 _]
                  tunnel: w582 -> [w600 _]
                  tunnel: w575 -> [_ w606]
                  tunnel: [TRUE FALSE] -> w574
                  tunnel: w577 -> [w595 w604]
                  tunnel: [w594 w604] -> w576
                  tunnel: [w593 path ""] -> w573
                  tunnel: [u16 3 ("Ctrl Mode") w602] -> w572
                  tunnel: ["Power (%)" "Power (%)"] -> w571
                  frame False {
                    n150 = Path To String(path=w593) -> (string=w597:string)
                    n151 = call "Device Launcher.vi"("Notifier Name"=w600, "Device Ports/IDs/Channels"=w596, "Device Engine Path"=w593) -> ()  [unwired: 11 in, 2 out]
                    n152 = Bundle By Name(cluster=w595, "Ctrl Mode"=u16 3, "Settings"=w596, "Ext Ctrl Path"=w597) -> (w594:T5)
                  }
                  frame True {
                    w602 = u16 1 ("Value")
                    n153 = property class="Ring (strict)"(reference=w606, "Value"=w602) -> ()  [unwired: 1 in, 2 out]
                  }
                }
              }
            }
            n154 = Index Array(array=w482, index=w454) -> (element=w483:T10)
            n155 = Bundle By Name(cluster=w483, "Ctrl Mode"=w463) -> (w481:T10)
            n156 = Replace Array Subset(array=w482, new element=w481, index=w454) -> (w479:T10[])
            n157 = Bundle By Name(cluster=w484, "Actions"=Laser_Power_Ctrl_Actions."Exit Loop", "Power Ctrl"=w479) -> (w485:T12)
            n158 = Type Cast(type=Laser_Power_Ctrl_Type."Direct" ("Control Mode"), x=w463) -> (*(type *) &x=w467:T17)
            n159 = Send Notification(notification=w485, notifier=w487) -> ()  [unwired: 1 in, 2 out]
            n160 = Format Into String(format string="%s", w467) -> (resulting string=w462:string)  [unwired: 2 in, 1 out]
            n161 = property class="Clust (strict)"(reference=w455) -> (reference out=w461:refnum<vi>, "Value"=w464:T1)  [unwired: 1 in, 1 out]
            n162 = Bundle By Name(cluster=w464, "Ctrl Status"=w462) -> (w460:T1)
            n163 = Replace Array Subset(array=w477, new element=w475, index=w454) -> (w474:T5[])
            n164 = property class="Clust (strict)"(reference=w461, "Value"=w460) -> ("Controls[]"=w458:refnum<vi>[])  [unwired: 1 in, 2 out]
            n165 = To More Generic Class(target class=w473, reference=w471) -> (generic class reference=w470:refnum<vi>)
            n166 = call "Laser Power Ctrl Enable Setup Controls.vi"("Enabled?"=w472, "Generic Class Ref"=w470, "VI Path"=w469) -> ()  [unwired: 13 in]
            n167 = call "Laser Power Ctrl Set Caption.vi"("Caption Text"=w459, "Setup Controls"=w458) -> ()  [unwired: 14 in]
          }
          event Value Change {
            w623 = refnum<vi> refnum  # Cluster
            w645 = refnum<vi> refnum  # Generic
            # "0: Direct\n1: AOTF\n2: External\n3: Ext + AOTF"
            n168 = event-data() -> ("CtlRef"=w620:refnum<vi>)  [unwired: 1 in, 2 out]
            n169 = To More Generic Class(target class=w645, reference=w620) -> (generic class reference=w644:refnum<vi>)
            n170 = property class="Bool (strict)"(reference=w620, "Value"=FALSE) -> ("Owner"=w624:refnum<vi>)  [unwired: 1 in, 2 out]
            n171 = call "Laser Power Ctrl Index from Name.vi"("Generic Class Ref"=w644) -> ("Index from Name"=w641:i32)  [unwired: 14 in]
            n172 = To More Specific Class(target class=w623, reference=w624) -> (specific class reference=w625:refnum<vi>)  [unwired: 1 in, 1 out]
            n173 = Index Array(array=w643, index=w641) -> (element=w642:T5)
            n174 = property class="Clust"(reference=w625) -> ("Controls[]"=w626:refnum<vi>[])  [unwired: 1 in, 2 out]
            n175 = Unbundle By Name(w642) -> ("Wavelength"=w629:u16, "Ext Ctrl Path"=w635:string, "Settings"=w633:string[])
            n176 = for {
              tunnel: w626 -> [w654] mode=indexing
              tunnel: [w651] -> w622
              tunnel: [w650] -> w621
              stop <- w651 stop-if-true
              n177 = property class="Ctl"(reference=w654) -> (reference out=w650:refnum<vi>, "Label.Text"=w653:string)  [unwired: 1 in, 1 out]
              n178 = Equal?(x=w653, y="Ext. Ctrl") -> (x = y?=w651:bool)
            }
            n179 = call "Laser Power Ctrl Wavelength to Notifier Name.vi"("Wavelength"=w629) -> ("Notifier Name"=w628:string)  [unwired: 13 in, 1 out]
            n180 = call "Device Manager Check if Running.vi"("Notifier Name"=w628) -> ("Running?"=w637:bool)  [unwired: 14 in]
            n181 = case shown="True" w637 {
              tunnel: w629 -> [w665 w671]
              tunnel: [w665 w671] -> w636
              tunnel: w635 -> [w664 w670]
              tunnel: [w664 w670] -> w634
              tunnel: w633 -> [w663 w669]
              tunnel: [w663 w669] -> w632
              tunnel: w628 -> [w662 w667]
              tunnel: [w662 w666] -> w631
              frame False {
              }
              frame True {
                n182 = call "Common Device Queue Messenger.vi"("Common Action"=Common_Device_Actions."Quit" ("Common Actions"), "Notifier Name"=w667) -> ("Notifier Name"=w666:string)  [unwired: 13 in]
              }
            }
            n183 = String To Path(string=w634) -> (path=w638:path)
            n184 = call "Laser Power Ctrl Ext Setup.vi"("Wavelength"=w636, "Previous Path"=w638, "Settings"=w632) -> ("Settings Out"=w627:string[], "Ext Ctrl Path"=w619:path, "Canceled?"=w630:bool)  [unwired: 10 in]
            n185 = Strip Path(path=w619) -> (name=w618:string)  [unwired: 1 out]
            n186 = case shown="False" w630 {
              tunnel: w619 -> [w655 _]
              tunnel: w627 -> [w658 _]
              tunnel: w631 -> [w660 _]
              tunnel: w642 -> [w657 w661]
              tunnel: [w656 w661] -> w640
              frame False {
                n187 = Path To String(path=w655) -> (string=w659:string)
                n188 = call "Device Launcher.vi"("Notifier Name"=w660, "Device Ports/IDs/Channels"=w658, "Device Engine Path"=w655) -> ()  [unwired: 11 in, 2 out]
                n189 = Bundle By Name(cluster=w657, "Settings"=w658, "Ext Ctrl Path"=w659) -> (w656:T5)
              }
              frame True {
              }
            }
            n190 = case shown="True" w622 {
              tunnel: w621 -> [_ w649]
              tunnel: w618 -> [_ w647]
              frame False {
              }
              frame True {
                n191 = To Variant(anything=w647) -> (Variant=w648:variant)
                n192 = property class="Ctl"(reference=w649, "Value"=w648) -> ()  [unwired: 1 in, 2 out]
              }
            }
            n193 = Replace Array Subset(array=w643, new element=w640, index=w641) -> (w639:T5[])
          }
          event Value Change {
            w679 = refnum<vi> refnum  # Generic
            n194 = event-data() -> ("CtlRef"=w681:refnum<vi>)  [unwired: 1 in, 1 out]
            n195 = property class="Bool (strict)"(reference=w681, "Value"=FALSE) -> ()  [unwired: 1 in, 2 out]
            n196 = To More Generic Class(target class=w679, reference=w681) -> (generic class reference=w678:refnum<vi>)
            n197 = call "Laser Power Ctrl Index from Name.vi"("Generic Class Ref"=w678) -> ("Index from Name"=w677:i32)  [unwired: 14 in]
            n198 = Index Array(array=w680, index=w677) -> (element=w675:T5)
            n199 = Unbundle By Name(w675) -> ("Wavelength"=w676:u16)
            n200 = call "Laser Power Ctrl Wavelength to Notifier Name.vi"("Wavelength"=w676) -> ("Notifier Name"=w673:string)  [unwired: 13 in, 1 out]
            n201 = call "Common Device Queue Messenger.vi"("Common Action"=Common_Device_Actions."Open Front Panel" ("Common Actions"), "Notifier Name"=w673) -> ()  [unwired: 13 in, 1 out]
          }
          event Value Change {
            # "Active: 2\nPower (%): 4\nPower Slider: 8"
            n202 = event-data() -> ("NewVal"=w683:T1, "OldVal"=w688:T1, "CtlRef"=w699:refnum<vi>)  [unwired: 1 in]
            n203 = Not Equal?(x=w683, y=w688) -> (x != y?=w690:T19)
            n204 = property class="Clust (strict)"(reference=w699) -> (reference out=w686:refnum<vi>, "Label.Text"=w692:string)  [unwired: 1 in, 1 out]
            n205 = Cluster To Array(cluster=w690) -> (array=w689:bool[])
            n206 = Boolean Array To Number(Boolean array=w689) -> (number=w687:u32)
            n207 = String Length(string=w692) -> (length=w698:i32)
            n208 = Subtract(x=w698, y=2) -> (x-y=w696:i32)
            n209 = String Subset(string=w692, offset (0)=w696) -> (substring=w693:string)  [unwired: 1 in]
            n210 = Scan From String(format string="%u", input string=w693, default 1=0) -> (output 1=w684:i32)  [unwired: 2 in, 3 out]
            n211 = case shown="4" w684 {
              tunnel: w683 -> [_ w701 w702 w703 w704 w705]
              frame Default {
              }
              frame 0 {
                n212 = local write "Power Ctrl 00"(w701) -> ()
              }
              frame 1 {
                n213 = local write "Power Ctrl 01"(w702) -> ()
              }
              frame 2 {
                n214 = local write "Power Ctrl 02"(w703) -> ()
              }
              frame 3 {
                n215 = local write "Power Ctrl 03"(w704) -> ()
              }
              frame 4 {
                n216 = local write "Power Ctrl 04"(w705) -> ()
              }
            }
            n217 = case shown="2" w687 {
              tunnel: w684 -> [_ w710 w724 w742]
              tunnel: w686 -> [_ w719 w736 w753]
              tunnel: w685 -> [_ w709 w722 w740]
              frame Default {
              }
              frame 2 {
                n218 = property class="Clust (strict)"(reference=w719) -> ("Value"=w718:T1)  [unwired: 1 in, 2 out]
                n219 = Unbundle By Name(w718) -> ("Wavelength (nm)"=w707:u16, "Active"=w706:bool)
                n220 = Get Notifier Status(notifier=w709) -> (notifier out=w717:refnum<notifier>, current notification=w715:T12)  [unwired: 1 in, 3 out]
                n221 = Unbundle By Name(w715) -> ("Power Ctrl"=w713:T10[])
                n222 = Index Array(array=w713, index=w710) -> (element=w714:T10)
                n223 = Bundle By Name(cluster=w714, "Active"=w706) -> (w712:T10)
                n224 = Replace Array Subset(array=w713, new element=w712, index=w710) -> (w711:T10[])
                n225 = Bundle By Name(cluster=w715, "Wavelength"=w707, "Power Ctrl"=w711, "Actions"=Laser_Power_Ctrl_Actions."Active") -> (w716:T12)
                n226 = Send Notification(notification=w716, notifier=w717) -> ()  [unwired: 1 in, 2 out]
              }
              frame 4 {
                n227 = property class="Clust (strict)"(reference=w736) -> (reference out=w735:refnum<vi>, "Value"=w734:T1)  [unwired: 1 in, 1 out]
                n228 = Unbundle By Name(w734) -> ("Power"=w723:dbl, "Wavelength (nm)"=w720:u16)
                n229 = To Unsigned Byte Integer(number=w723) -> (unsigned 8bit integer=w733:u8)
                n230 = Get Notifier Status(notifier=w722) -> (notifier out=w731:refnum<notifier>, current notification=w729:T12)  [unwired: 1 in, 3 out]
                n231 = Bundle By Name(cluster=w734, "Power Slider"=w733) -> (w732:T1)
                n232 = Unbundle By Name(w729) -> ("Power Ctrl"=w727:T10[])
                n233 = property class="Clust (strict)"(reference=w735, "Value"=w732) -> ()  [unwired: 1 in, 2 out]
                n234 = Index Array(array=w727, index=w724) -> (element=w728:T10)
                n235 = Bundle By Name(cluster=w728, "Power"=w723) -> (w726:T10)
                n236 = Replace Array Subset(array=w727, new element=w726, index=w724) -> (w725:T10[])
                n237 = Bundle By Name(cluster=w729, "Wavelength"=w720, "Power Ctrl"=w725, "Actions"=Laser_Power_Ctrl_Actions."Power Adj") -> (w730:T12)
                n238 = Send Notification(notification=w730, notifier=w731) -> ()  [unwired: 1 in, 2 out]
              }
              frame 8 {
                n239 = property class="Clust (strict)"(reference=w753) -> (reference out=w752:refnum<vi>, "Value"=w751:T1)  [unwired: 1 in, 1 out]
                n240 = Unbundle By Name(w751) -> ("Power Slider"=w741:u8, "Wavelength (nm)"=w738:u16)
                n241 = To Double Precision Float(number=w741) -> (double precision float=w737:dbl)
                n242 = Get Notifier Status(notifier=w740) -> (notifier out=w749:refnum<notifier>, current notification=w747:T12)  [unwired: 1 in, 3 out]
                n243 = Bundle By Name(cluster=w751, "Power"=w737) -> (w750:T1)
                n244 = Unbundle By Name(w747) -> ("Power Ctrl"=w745:T10[])
                n245 = property class="Clust (strict)"(reference=w752, "Value"=w750) -> ()  [unwired: 1 in, 2 out]
                n246 = Index Array(array=w745, index=w742) -> (element=w746:T10)
                n247 = Bundle By Name(cluster=w746, "Power"=w737) -> (w744:T10)
                n248 = Replace Array Subset(array=w745, new element=w744, index=w742) -> (w743:T10[])
                n249 = Bundle By Name(cluster=w747, "Wavelength"=w738, "Power Ctrl"=w743, "Actions"=Laser_Power_Ctrl_Actions."Power Adj") -> (w748:T12)
                n250 = Send Notification(notification=w748, notifier=w749) -> ()  [unwired: 1 in, 2 out]
              }
            }
          }
          event "Manual Laser Ctrl.": Value Change {
            n251 = event-data() -> ("NewVal"=w757:bool)  [unwired: 1 in]
            n252 = Select(t=Laser_Power_Ctrl_Actions."All Active On" ("Actions"), s=w757, f=Laser_Power_Ctrl_Actions."All Active Off") -> (s? t:f=w755:T11)
            n253 = Get Notifier Status(notifier=w760) -> (notifier out=w761:refnum<notifier>, current notification=w759:T12)  [unwired: 1 in, 3 out]
            n254 = Bundle By Name(cluster=w759, "Actions"=w755) -> (w754:T12)
            n255 = Send Notification(notification=w754, notifier=w761) -> ()  [unwired: 1 in, 2 out]
          }
          event "Power Ctrl Setup": Value Change {
            n256 = event-data() -> ("NewVal"=w768:bool)  [unwired: 1 in]
            n257 = Select(t=enum32{"Power Adjust", "Setup"}."Setup" ("Tab Control"), s=w768, f=enum32{"Power Adjust", "Setup"}."Power Adjust" ("Tab Control")) -> (s? t:f=→"Tab Control":enum32{"Power Adjust", "Setup"})
          }
          event "Quit": Value Change {
            n258 = event-data() -> ("NewVal"=w786:bool)  [unwired: 1 in]
            n259 = Get Notifier Status(notifier=w785) -> (notifier out=w783:refnum<notifier>, current notification=w784:T12)  [unwired: 1 in, 3 out]
            n260 = Bundle By Name(cluster=w784, "Actions"=Laser_Power_Ctrl_Actions."Quit") -> (w781:T12)
            n261 = Read from Text File(file (use dialog)=w770) -> (text=w780:string, error out=w779:errorcluster)  [unwired: 3 in, 2 out]
            n262 = Initialize Array(T5 {"Wavelength"=999, "Ctrl Mode"=999, "Ext Ctrl Path"="", "Settings"=[]} ("Power Ctrl Settings"), 5 ("dimension size")) -> (w774:T5[])
            n263 = Unflatten From JSON(JSON string=w780, type and defaults=w774, error in (no error)=w779) -> (value=w775:T5[], error out=w776:errorcluster)  [unwired: 4 in]
            n264 = Send Notification(notification=w781, notifier=w783) -> ()  [unwired: 1 in, 2 out]
            n265 = case shown="Error" w776 {
              tunnel: w775 -> [w796 _]
              tunnel: [w796 w797] -> w773
              tunnel: w774 -> [_ w797]
              frame No Error {
              }
              frame Error {
              }
            }
            n266 = Not Equal?(x=w771, y=w773) -> (x != y?=w772:bool)
            n267 = case shown="True" w772 {
              tunnel: w771 -> [_ w787]
              tunnel: w770 -> [_ w788]
              frame False {
              }
              frame True {
                n268 = Two Button Dialog(message="Save current settings as default values?", 1:"No" ("F button name (\"Cancel\")"), 2:"Yes" ("T button name (\"OK\")")) -> (T button?=w789:bool)
                n269 = case shown="True" w789 {
                  tunnel: w787 -> [_ w794]
                  tunnel: w788 -> [_ w793]
                  frame False {
                  }
                  frame True {
                    n270 = Flatten To JSON(anything=w794) -> (JSON string=w795:string)  [unwired: 2 in, 1 out]
                    n271 = Write to Text File(file (use dialog)=w793, text=w795) -> ()  [unwired: 2 in, 3 out]
                  }
                }
              }
            }
          }
        }
      }
      n272 = while {
        tunnel: w232 -> [w260]
        shift-right: [w252] -> _
        shift-left: FALSE -> [w253]
        tunnel: w218 -> [w251]
        tunnel: w219 -> [w250]
        stop <- w257 stop-if-true
        n273 = Wait on Notification(notifier=w260, ignore previous (F)=TRUE) -> (notifier out=w254:refnum<notifier>, notification=w255:T12)  [unwired: 2 in, 2 out]
        n274 = Unbundle By Name(w255) -> ("Actions"=w256:T11)
        n275 = Equal?(x=w256, y=Laser_Power_Ctrl_Actions."Quit") -> (x = y?=w257:bool)
        n276 = case shown="\"Power Adj\"" w256 {
          tunnel: w255 -> [_ w271 w317 w349 w384 _]
          tunnel: w254 -> [_ _ _ _ _ w420]
          tunnel: w253 -> [w261 w266 _ _ w379 w419]
          tunnel: [w261 w268 TRUE FALSE w381 w419] -> w252
          tunnel: w251 -> [_ w264 w314 w346 w377 _]
          tunnel: w250 -> [_ w262 w316 w348 w375 _]
          frame "Exit Loop", Default {
          }
          frame "Active" {
            # "0: Direct\n1: AOTF\n2: External"
            n277 = Unbundle By Name(w271) -> ("Power Ctrl"=w270:T10[], "Wavelengths"=w272:u16[], "Wavelength"=w265:u16)
            n278 = Search 1D Array(1D array=w272, element=w265) -> (index of element=w263:i32)  [unwired: 1 in]
            n279 = Index Array(array=w270, index=w263) -> (element=w267:T10)
            n280 = Less Than 0?(x=w263) -> (x < 0?=w269:bool)
            n281 = case shown="False" w269 {
              tunnel: w266 -> [w273 w311]
              tunnel: [w273 w311] -> w268
              tunnel: w267 -> [w281 _]
              tunnel: w265 -> [w275 _]
              tunnel: w264 -> [w279 _]
              tunnel: w263 -> [w278 _]
              tunnel: w262 -> [w276 _]
              frame False {
                n282 = Unbundle By Name(w281) -> ("Ctrl Mode"=w280:u16, "Active"=w274:bool)
                n283 = Index Array(array=w279, index=w278) -> (element=w277:string)
                n284 = case shown="3" w280 {
                  tunnel: w274 -> [_ w283 w291 w296 w300]
                  tunnel: w277 -> [_ w285 _ _ _]
                  tunnel: w276 -> [_ _ w290 _ w307]
                  tunnel: w275 -> [_ _ w289 w294 w302]
                  tunnel: w273 -> [_ w284 _ w297 w301]
                  frame Default {
                  }
                  frame 0 {
                    n285 = And(x=w283, y=w284) -> (x .and. y?=w282:bool)
                    n286 = call "Laser Messenger.vi"("Notifier Name"=w285, "Action"=Laser_Actions."Set On/Off", "Emission On/Off"=w282) -> ()  [unwired: 7 in, 6 out]
                  }
                  frame 1 {
                    n287 = Format Into String(format string="%u", w289) -> (resulting string=w288:string)  [unwired: 2 in, 1 out]
                    n288 = call "AOTF Messenger.vi"("AOTF Notifier Name"=w290, "AOTF Action"=AOTF_Actions."Line On/Off", "Wavelength (nm)"=w288, "Line On/Off"=w291) -> ()  [unwired: 6 in, 6 out]
                  }
                  frame 2 {
                    n289 = call "Laser Power Ctrl Wavelength to Notifier Name.vi"("Wavelength"=w294) -> ("Notifier Name"=w299:string, "Wavelength"=w293:string)  [unwired: 13 in]
                    n290 = And(x=w296, y=w297) -> (x .and. y?=w298:bool)
                    n291 = call "External Pwr Ctrl Messenger.vi"("Notifier Name"=w299, "Actions"=External_Power_Actions."Line On/Off", "Wavelength"=w293, "Line On/Off"=w298) -> ()  [unwired: 12 in]
                  }
                  frame 3 {
                    n292 = call "Laser Power Ctrl Wavelength to Notifier Name.vi"("Wavelength"=w302) -> ("Notifier Name"=w306:string, "Wavelength"=w303:string)  [unwired: 13 in]
                    n293 = And(x=w300, y=w301) -> (x .and. y?=w305:bool)
                    n294 = Format Into String(format string="%u", w302) -> (resulting string=w309:string)  [unwired: 2 in, 1 out]
                    n295 = call "External Pwr Ctrl Messenger.vi"("Notifier Name"=w306, "Actions"=External_Power_Actions."Line On/Off", "Wavelength"=w303, "Line On/Off"=w305) -> ()  [unwired: 12 in]
                    n296 = call "AOTF Messenger.vi"("AOTF Notifier Name"=w307, "AOTF Action"=AOTF_Actions."Line On/Off", "Wavelength (nm)"=w309, "Line On/Off"=w300) -> ()  [unwired: 6 in, 6 out]
                  }
                }
              }
              frame True {
              }
            }
          }
          frame "All Active On" {
            # "0: Direct\n1: AOTF\n2: External\n3: Ext + AOTF"
            n297 = Unbundle By Name(w317) -> ("Power Ctrl"=w313:T10[], "Wavelengths"=w312:u16[])
            n298 = for {
              tunnel: w316 -> [w323]
              tunnel: w314 -> [w320] mode=indexing
              tunnel: w313 -> [w319] mode=indexing
              tunnel: w312 -> [w318] mode=indexing
              n299 = Unbundle By Name(w319) -> ("Ctrl Mode"=w322:u16, "Active"=w321:bool)
              n300 = case shown="3" w322 {
                tunnel: w321 -> [_ w325 _ w331 w336]
                tunnel: w320 -> [_ w326 _ _ _]
                tunnel: w323 -> [_ _ w329 _ w341]
                tunnel: w318 -> [_ _ _ w332 w337]
                frame Default {
                }
                frame 0 {
                  n301 = call "Laser Messenger.vi"("Notifier Name"=w326, "Action"=Laser_Actions."Set On/Off", "Emission On/Off"=w325, "Exit While Busy (F)?"=FALSE) -> ()  [unwired: 6 in, 6 out]
                }
                frame 1 {
                  n302 = call "AOTF Messenger.vi"("AOTF Notifier Name"=w329, "AOTF Action"=AOTF_Actions."Blank", "Beam Blank"=FALSE) -> ()  [unwired: 7 in, 6 out]
                }
                frame 2 {
                  n303 = call "Laser Power Ctrl Wavelength to Notifier Name.vi"("Wavelength"=w332) -> ("Notifier Name"=w335:string, "Wavelength"=w333:string)  [unwired: 13 in]
                  n304 = call "External Pwr Ctrl Messenger.vi"("Notifier Name"=w335, "Actions"=External_Power_Actions."Line On/Off", "Wavelength"=w333, "Line On/Off"=w331) -> ()  [unwired: 12 in]
                }
                frame 3 {
                  n305 = call "Laser Power Ctrl Wavelength to Notifier Name.vi"("Wavelength"=w337) -> ("Notifier Name"=w340:string, "Wavelength"=w338:string)  [unwired: 13 in]
                  n306 = call "AOTF Messenger.vi"("AOTF Notifier Name"=w341, "AOTF Action"=AOTF_Actions."Blank", "Beam Blank"=FALSE) -> ()  [unwired: 7 in, 6 out]
                  n307 = call "External Pwr Ctrl Messenger.vi"("Notifier Name"=w340, "Actions"=External_Power_Actions."Line On/Off", "Wavelength"=w338, "Line On/Off"=w336) -> ()  [unwired: 12 in]
                }
              }
            }
          }
          frame "All Active Off" {
            # "0: Direct\n1: AOTF\n2: External\n3: Ext + AOTF"
            n308 = Unbundle By Name(w349) -> ("Power Ctrl"=w345:T10[], "Wavelengths"=w344:u16[])
            n309 = for {
              tunnel: w348 -> [w355]
              tunnel: w346 -> [w353] mode=indexing
              tunnel: w345 -> [w352] mode=indexing
              tunnel: w344 -> [w351] mode=indexing
              n310 = Unbundle By Name(w352) -> ("Ctrl Mode"=w354:u16)
              n311 = case shown="3" w354 {
                tunnel: FALSE -> [_ w356 _ w362 w370]
                tunnel: w353 -> [_ w357 _ _ _]
                tunnel: w355 -> [_ _ w360 _ w367]
                tunnel: w351 -> [_ _ _ w363 w371]
                frame Default {
                }
                frame 0 {
                  n312 = call "Laser Messenger.vi"("Notifier Name"=w357, "Action"=Laser_Actions."Set On/Off", "Emission On/Off"=w356) -> ()  [unwired: 7 in, 6 out]
                }
                frame 1 {
                  n313 = call "AOTF Messenger.vi"("AOTF Notifier Name"=w360, "AOTF Action"=AOTF_Actions."Blank", "Beam Blank"=TRUE ("Beam Blank 2")) -> ()  [unwired: 7 in, 6 out]
                }
                frame 2 {
                  n314 = call "Laser Power Ctrl Wavelength to Notifier Name.vi"("Wavelength"=w363) -> ("Notifier Name"=w366:string, "Wavelength"=w364:string)  [unwired: 13 in]
                  n315 = call "External Pwr Ctrl Messenger.vi"("Notifier Name"=w366, "Actions"=External_Power_Actions."Line On/Off", "Wavelength"=w364, "Line On/Off"=w362) -> ()  [unwired: 12 in]
                }
                frame 3 {
                  n316 = call "Laser Power Ctrl Wavelength to Notifier Name.vi"("Wavelength"=w371) -> ("Notifier Name"=w374:string, "Wavelength"=w372:string)  [unwired: 13 in]
                  n317 = call "AOTF Messenger.vi"("AOTF Notifier Name"=w367, "AOTF Action"=AOTF_Actions."Blank", "Beam Blank"=TRUE ("Beam Blank 2")) -> ()  [unwired: 7 in, 6 out]
                  n318 = call "External Pwr Ctrl Messenger.vi"("Notifier Name"=w374, "Actions"=External_Power_Actions."Line On/Off", "Wavelength"=w372, "Line On/Off"=w370) -> ()  [unwired: 12 in]
                }
              }
            }
          }
          frame "Power Adj" {
            # "0: Direct\n1: AOTF\n2: External"
            n319 = Unbundle By Name(w384) -> ("Power Ctrl"=w383:T10[], "Wavelengths"=w385:u16[], "Wavelength"=w378:u16)
            n320 = Search 1D Array(1D array=w385, element=w378) -> (index of element=w376:i32)  [unwired: 1 in]
            n321 = Index Array(array=w383, index=w376) -> (element=w380:T10)
            n322 = Less Than 0?(x=w376) -> (x < 0?=w382:bool)
            n323 = case shown="False" w382 {
              tunnel: w379 -> [w392 w418]
              tunnel: [w392 w418] -> w381
              tunnel: w380 -> [w394 _]
              tunnel: w378 -> [w387 _]
              tunnel: w377 -> [w391 _]
              tunnel: w376 -> [w390 _]
              tunnel: w375 -> [w388 _]
              frame False {
                n324 = Unbundle By Name(w394) -> ("Ctrl Mode"=w393:u16, "Power"=w386:dbl)
                n325 = Index Array(array=w391, index=w390) -> (element=w389:string)
                n326 = case shown="3" w393 {
                  tunnel: w389 -> [_ w396 _ _ _]
                  tunnel: w388 -> [_ _ w402 _ w410]
                  tunnel: w387 -> [_ _ w399 w405 w411]
                  tunnel: w386 -> [_ w395 w401 w404 w409]
                  frame Default {
                  }
                  frame 0 {
                    n327 = call "Laser Messenger.vi"("Notifier Name"=w396, "Action"=Laser_Actions."Set Power", "Power (mW)"=w395) -> ()  [unwired: 7 in, 6 out]
                  }
                  frame 1 {
                    n328 = Format Into String(format string="%u", w399) -> (resulting string=w398:string)  [unwired: 2 in, 1 out]
                    n329 = call "AOTF Messenger.vi"("AOTF Notifier Name"=w402, "AOTF Action"=AOTF_Actions."Set Power", "Wavelength (nm)"=w398, "Power (%)"=w401) -> ()  [unwired: 6 in, 6 out]
                  }
                  frame 2 {
                    n330 = call "Laser Power Ctrl Wavelength to Notifier Name.vi"("Wavelength"=w405) -> ("Notifier Name"=w408:string, "Wavelength"=w406:string)  [unwired: 13 in]
                    n331 = call "External Pwr Ctrl Messenger.vi"("Notifier Name"=w408, "Actions"=External_Power_Actions."Set Power", "Wavelength"=w406, "Power (%)"=w404) -> ()  [unwired: 12 in]
                  }
                  frame 3 {
                    n332 = call "Laser Power Ctrl Wavelength to Notifier Name.vi"("Wavelength"=w411) -> ("Notifier Name"=w417:string, "Wavelength"=w415:string)  [unwired: 13 in]
                    n333 = Format Into String(format string="%u", w411) -> (resulting string=w412:string)  [unwired: 2 in, 1 out]
                    n334 = call "External Pwr Ctrl Messenger.vi"("Notifier Name"=w417, "Actions"=External_Power_Actions."Set Power", "Wavelength"=w415, "Power (%)"=w409) -> ()  [unwired: 12 in]
                    n335 = call "AOTF Messenger.vi"("AOTF Notifier Name"=w410, "AOTF Action"=AOTF_Actions."Set Power", "Wavelength (nm)"=w412, "Power (%)"=w409) -> ()  [unwired: 6 in, 6 out]
                  }
                }
              }
              frame True {
              }
            }
          }
          frame "Quit" {
            n336 = Release Notifier(notifier=w420) -> ()  [unwired: 2 in, 3 out]
          }
        }
      }
    }
    frame True {
    }
  }
